vi "SubVI_IntakePositions_teleop.vi"() -> ()   [LabVIEW 2017]
uses:
  <vilib>/Rock Robotics/WPI/Utilities/WPI_GetSetVariantRefNum.vi
  <vilib>/Rock Robotics/Network Tables/NT Read Number.vi
  <vilib>/Rock Robotics/Network Tables/NT Write Number.vi
panel:
  out "IntakePos":dbl
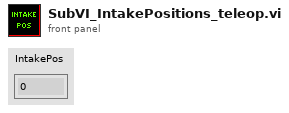
[diagram p1: front panel]
types:
  T1 = typedef "WPI_JoystickDevRef.ctl" = cluster{"Device":T2}
  T2 = typedef "WPI_JoystickDeviceEnum.ctl" = enum16{"USB 0", "USB 1", "USB 2", "USB 3", "USB 4", "USB 5"}
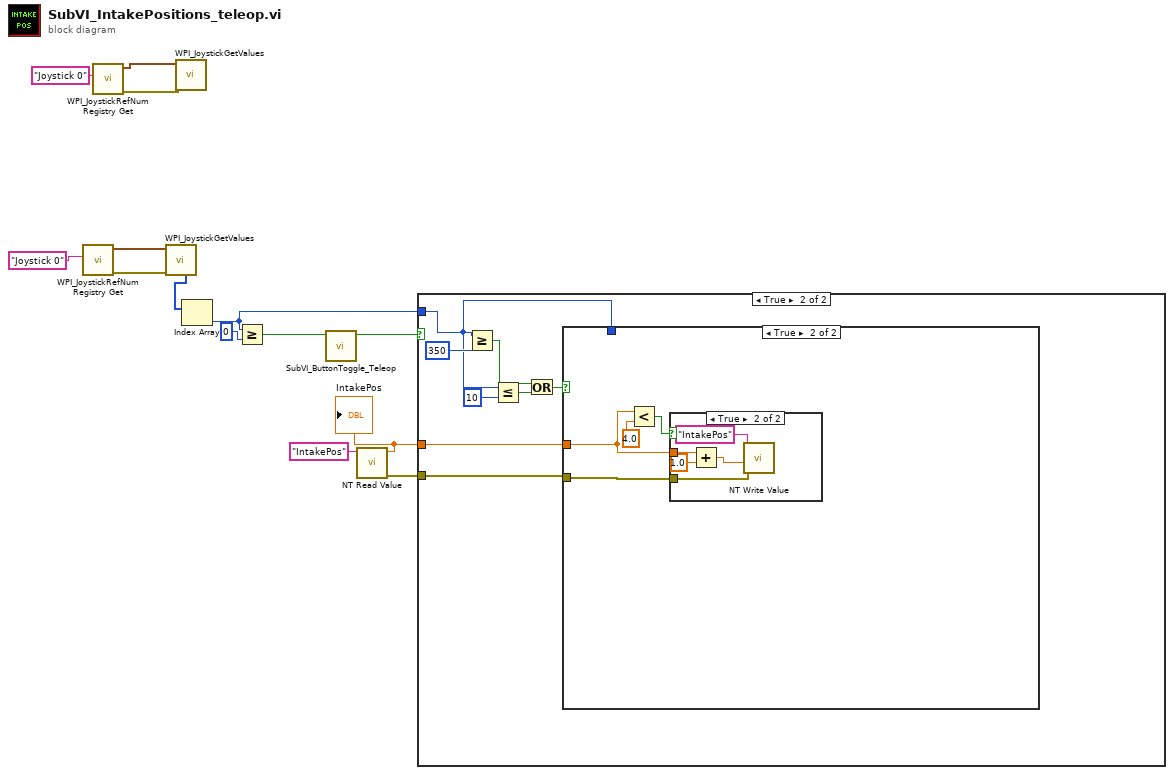
[diagram p0: block diagram]
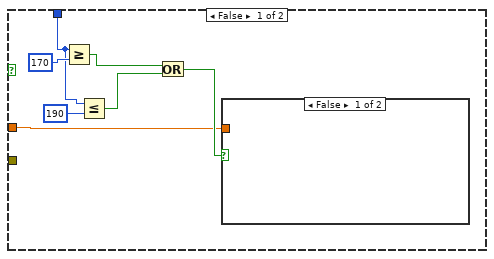
[diagram p3: hidden frame]
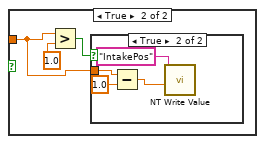
[diagram p4: hidden frame]
diagram:
  n1 = call <vilib>:"WPI_JoystickRefNum Registry Get.vi"("refnum name"="Joystick 0") -> ("error out"=w8:errorcluster, "JoystickDevRef"=w7:T1)  [unwired: 9 in]
  n2 = call <vilib>:"WPI_JoystickRefNum Registry Get.vi"("refnum name"="Joystick 0") -> ("error out"=w11:errorcluster, "JoystickDevRef"=w10:T1)  [unwired: 9 in]
  n3 = call <vilib>:"WPI_JoystickGetValues.vi"("error in (no error)"=w8, "JoystickDevRef"=w7) -> ("POVs"=w13:i16[])  [unwired: 5 in, 4 out]
  n4 = call <vilib>:"WPI_JoystickGetValues.vi"("error in (no error)"=w11, "JoystickDevRef"=w10) -> ()  [unwired: 5 in, 5 out]
  n5 = Index Array(array=w13) -> (element=w6:i16)  [unwired: 1 in]
  n6 = Greater Or Equal?(x=w6, y=i16 0) -> (x >= y?=w2:bool)
  n7 = call "SubVI_ButtonToggle_Teleop.vi"("Boolean in"=w2) -> ("Boolean out"=w1:bool)  [unwired: 10 in]
  n8 = call-poly <vilib>:"NT Read Value.vi"("Name"="IntakePos") -> ("error out"=w4:errorcluster, "Numeric"=w3:dbl)  [unwired: 9 in]
  "IntakePos" <- w3
  n9 = case shown="True" w1 {
    tunnel: w6 -> [_ w17]
    tunnel: w4 -> [_ w16]
    tunnel: w3 -> [_ w15]
    frame False {
    }
    frame True {
      n10 = Greater Or Equal?(x=w17, y=i16 350) -> (x >= y?=w21:bool)
      n11 = Less Or Equal?(x=w17, y=i16 10) -> (x <= y?=w19:bool)
      n12 = Or(x=w21, y=w19) -> (x .or. y?=w18:bool)
      n13 = case shown="True" w18 {
        tunnel: w15 -> [w23 w40]
        tunnel: w16 -> [_ w37]
        tunnel: w17 -> [w25 _]
        frame False {
          n14 = Greater Or Equal?(x=w25, y=i16 170) -> (x >= y?=w28:bool)
          n15 = Less Or Equal?(x=w25, y=i16 190) -> (x <= y?=w26:bool)
          n16 = Or(x=w28, y=w26) -> (x .or. y?=w24:bool)
          n17 = case shown="False" w24 {
            tunnel: w23 -> [_ w30]
            frame False {
            }
            frame True {
              n18 = Greater?(x=w30, y=1.0) -> (0:w31:bool)
              n19 = case shown="True" w31 {
                tunnel: w30 -> [_ w33]
                frame False {
                }
                frame True {
                  n20 = Subtract(x=w33, y=1.0) -> (x-y=w34:dbl)
                  n21 = call-poly <vilib>:"NT Write Value.vi"("Numeric"=w34, "Name"="IntakePos") -> ()  [unwired: 9 in, 1 out]
                }
              }
            }
          }
        }
        frame True {
          n22 = Less?(x=w40, y=4.0) -> (x < y?=w38:bool)
          n23 = case shown="True" w38 {
            tunnel: w40 -> [_ w45]
            tunnel: w37 -> [_ w41]
            frame False {
            }
            frame True {
              n24 = Add(x=w45, y=1.0) -> (x+y=w42:dbl)
              n25 = call-poly <vilib>:"NT Write Value.vi"("error in"=w41, "Numeric"=w42, "Name"="IntakePos") -> ()  [unwired: 8 in, 1 out]
            }
          }
        }
      }
    }
  }
